vi "OpenCV_LabVIEW_HueConvert.vi"() -> (2 "OpenCV to LV":dbl, 3 "LV to OpenCV":dbl)   [LabVIEW 2020]
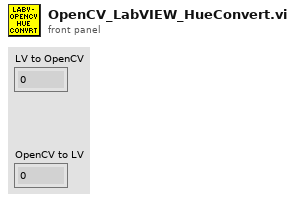
[diagram p1: front panel]
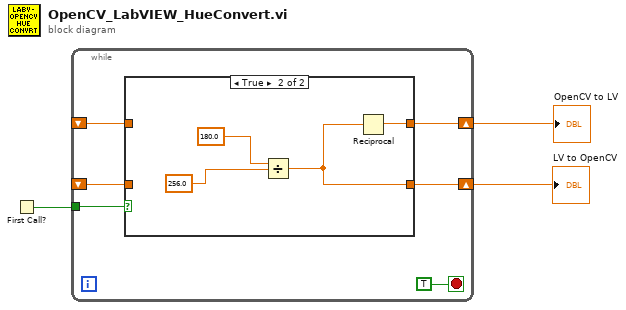
[diagram p0: block diagram]
diagram:
  n1 = First Call?() -> (First Call?: T/F=w1:bool)
  n2 = while {
    shift-right: [w9] -> w3
    shift-left: _ -> [w4]
    shift-right: [w8] -> w2
    shift-left: _ -> [w5]
    tunnel: w1 -> [w6]
    stop <- TRUE stop-if-true
    n3 = case shown="True" w6 {
      tunnel: [w10 w15] -> w9
      tunnel: [w11 w14] -> w8
      tunnel: w5 -> [w11 _]
      tunnel: w4 -> [w10 _]
      frame False {
      }
      frame True {
        n4 = Divide(x=180.0, y=256.0) -> (x/y=w15:dbl)
        n5 = Reciprocal(x=w15) -> (1/x=w14:dbl)
      }
    }
  }
  "LV to OpenCV" <- w3
  "OpenCV to LV" <- w2
